vi "Read Digital Outputs.vi"(8 "error in (no error)":errorcluster, 11 "Stage Actor.lvlib:Stage.lvclass":refnum<class "Stage.lvclass">) -> (0 "error out":errorcluster, 3 "Stage Actor.lvlib:Stage.lvclass":refnum<class "Stage.lvclass">)   [LabVIEW 2018, in "Stage Actor.lvlib" / "Stage.lvclass"]
uses:
  Stage.lvclass
  C:/Program Files/National Instruments/LabVIEW 2018/vi.lib/ActorFramework/Actor/Actor.lvclass
  <vilib>/ActorFramework/Actor/Actor.lvclass/Actor.ctl
  Stage.lvclass/Stage.ctl
  <instrlib>/Zaber A Series/Zaber A Series.lvlib
  <vilib>/ActorFramework/Actor/Actor.lvclass
  ADM/Main Messages/Set Print Msg/Set Print Msg.lvclass
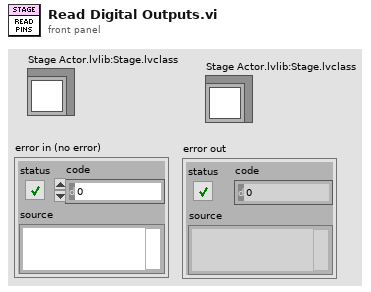
[diagram p1: front panel]
types:
  T1 = cluster{"Digital Output Pins[0]":bool, "Digital Output Pins[1]":bool, "Digital Output Pins[2]":bool, "Digital Output Pins[3]":bool, "Digital Output Pins[4]":bool, "Digital Output Pins[5]":bool, "Digital Output Pins[6]":bool, "Digital Output Pins[7]":bool, "Digital Output Pins[8]":bool}
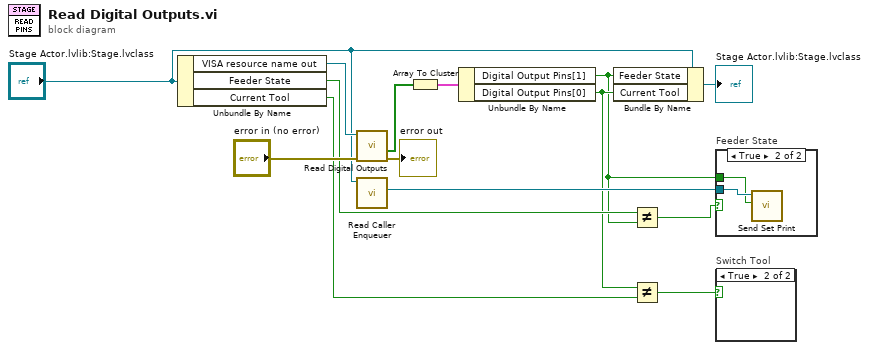
[diagram p0: block diagram]
diagram:
  n1 = Unbundle By Name("Stage Actor.lvlib:Stage.lvclass") -> ("VISA resource name out"=w14:refnum<visa-resource-name>, "Feeder State"=w4:bool, "Current Tool"=w3:bool)
  n2 = call <instrlib>:"Read Digital Outputs.vi"("error in (no error)"="error in (no error)", "VISA resource name"=w14) -> ("error out"=→"error out":errorcluster, "Digital Output Pins"=w12:bool[])  [unwired: 7 in, 1 out]
  n3 = call <vilib>:"Read Caller Enqueuer.vi"("Actor"="Stage Actor.lvlib:Stage.lvclass") -> ("Caller Enqueuer"=w10:refnum<class "Message Enqueuer.lvclass">)  [unwired: 10 in]
  n4 = Array To Cluster(array=w12) -> (cluster=w13:T1)
  n5 = Unbundle By Name(w13) -> ("Digital Output Pins[1]"=w1:bool, "Digital Output Pins[0]"=w2:bool)
  n6 = Bundle By Name(cluster="Stage Actor.lvlib:Stage.lvclass", "Feeder State"=w1, "Current Tool"=w2) -> (→"Stage Actor.lvlib:Stage.lvclass":refnum<class "Stage.lvclass">)
  n7 = Not Equal?(x=w4, y=w1) -> (x != y?=w5:bool)
  n8 = Not Equal?(x=w2, y=w3) -> (x != y?=w6:bool)
  n9 = case "Feeder State" shown="True" w5 {
    tunnel: w10 -> [_ w16]
    tunnel: w1 -> [_ w15]
    frame False {
    }
    frame True {
      n10 = call "Send Set Print.vi"("On?"=w15, "Message Enqueuer in"=w16) -> ()  [unwired: 8 in, 2 out]
    }
  }
  n11 = case "Switch Tool" shown="True" w6 {
    frame False {
    }
    frame True {
    }
  }
